vi "p1.vi"() -> ()   [LabVIEW 2021, in "d7.lvlib"]
uses:
  d7.lvlib
  dir/dir.lvclass
  AOC/AOC.lvlib
panel:
  out "Answer":i64=1141028
  in  "Example":string="$ cd /\n$ ls\ndir a\n14848514 b.txt\n8504156 c.dat\ndir d\n$ cd a\n$ ls\ndir e\n29116 f\n2557 g\n62596 h.lst\n$ cd e\n$ ls\n584 i\n$ cd ..\n$ cd ..\n$ cd d\n$ ls\n4060174 j\n8033020 d.log\n5626152 d.ext\n7214296 k"
  in  "Example":bool
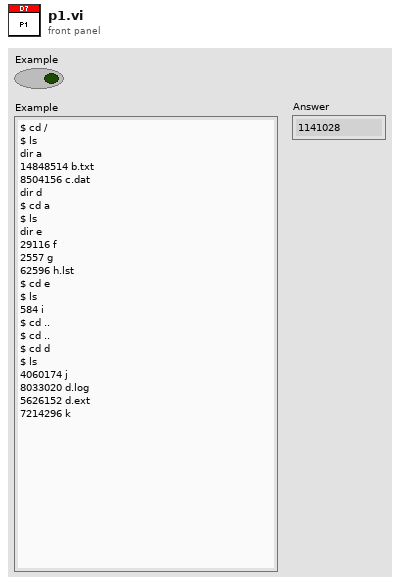
[diagram p1: front panel]
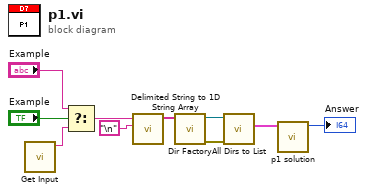
[diagram p0: block diagram]
diagram:
  n1 = call "Get Input.vi"() -> ("Input"=w10:string)  [unwired: 11 in]
  n2 = Select(t="Example", s="Example", f=w10) -> (s? t:f=w9:string)
  n3 = call <vilib>:"Delimited String to 1D String Array.vi"("delimiter"="\n", "delimited string"=w9) -> ("string array"=w3:string[])  [unwired: 9 in]
  n4 = call "Dir Factory.vi"("Commands"=w3) -> ("error out"=w1:errorcluster, "dir out"=w2:refnum<class "dir.lvclass">)  [unwired: 9 in]
  n5 = call-dynamic "All Dirs to List.vi"("error in (no error)"=w1, "dir in"=w2) -> ("Dir List"=w5:cluster{"Name":string, "Size":i64}[])  [unwired: 7 in, 2 out]
  n6 = call "p1 solution.vi"("Dir List"=w5) -> ("Size"=→"Answer":i64)  [unwired: 10 in]
